vi "get_file_name_base.vi"(8 "error in (no error)":errorcluster, 11 "GenericComponent in":refnum<class "GenericComponent.lvclass">) -> (0 "error out":errorcluster, 2 "file name base":string, 3 "GenericComponent out":refnum<class "GenericComponent.lvclass">)   [LabVIEW 2010, in "GenericComponent.lvclass"]
uses:
  GenericComponent.lvclass
  class_data.vi
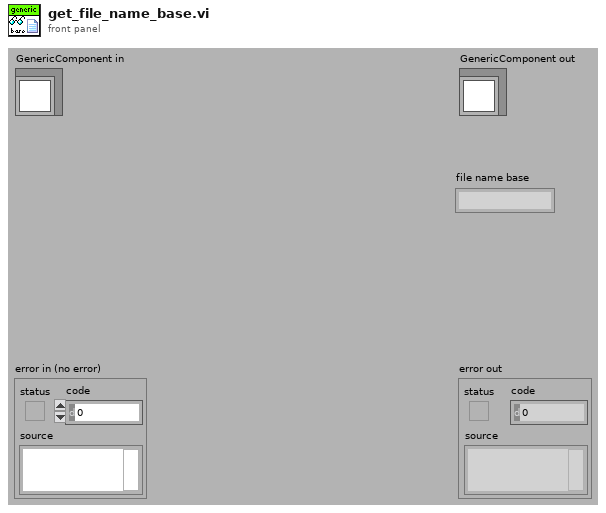
[diagram p1: front panel]
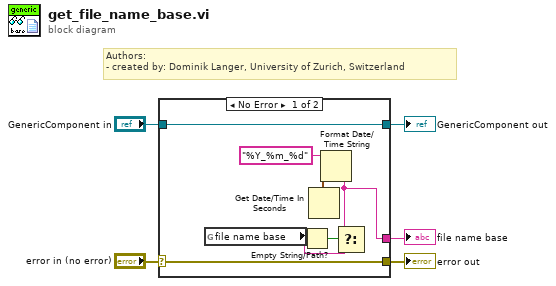
[diagram p0: block diagram]
diagram:
  # "Authors: \n- created by: Dominik Langer, University of Zurich, Switzerland"
  n1 = case shown="No Error" "error in (no error)" {
    selector: "error in (no error)" -> [w11 w14]
    tunnel: [w11 w14] -> w4
    tunnel: [w12 w13] -> w2
    tunnel: "GenericComponent in" -> [w12 w13]
    tunnel: [w6 _] -> w1
    frame No Error {
      n2 = global read "class_data.vi" "file name base"() -> (w7:string)
      n3 = Empty String/Path?(string/path=w7) -> (empty?=w8:bool)
      n4 = Get Date/Time In Seconds() -> (seconds since 1Jan1904=w9:timestamp)
      n5 = Format Date/Time String(time format string (%c)="%Y_%m_%d", seconds (now)=w9) -> (date/time string=w6:string)  [unwired: 1 out]
      n6 = Select(t=w6, s=w8, f=w7) -> ()  [unwired: 1 out]
    }
    frame Error {
    }
  }
  "error out" <- w4
  "GenericComponent out" <- w2
  "file name base" <- w1
